vi "SumTwoh.vi"(0 "h1":dbl[](array[numeric]) format="%.2f", 1 "delay1":i32, 2 "h2":dbl[](array[numeric]) format="%.2f", 3 "delay2":i32) -> (4 "delay out":i32, 5 "upper":dbl[](array[numeric]) format="%.2f", 6 "h sum":dbl[](array[numeric]) format="%.2f", 7 "lower":dbl[](array[numeric]) format="%.2f")   [LabVIEW 2022 SP3]
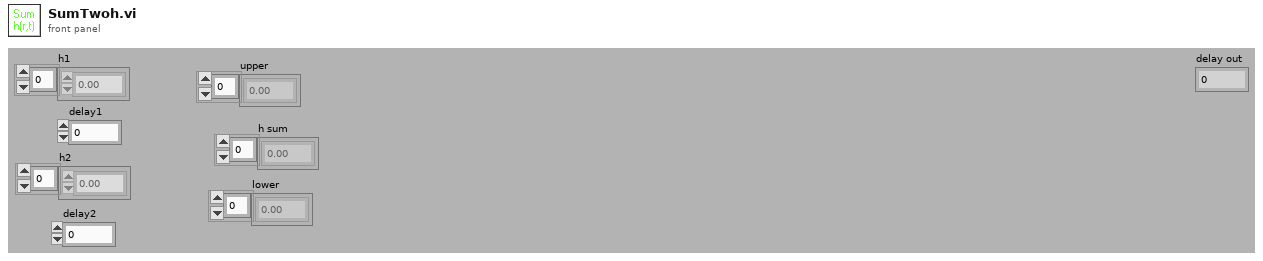
[diagram p1: front panel]
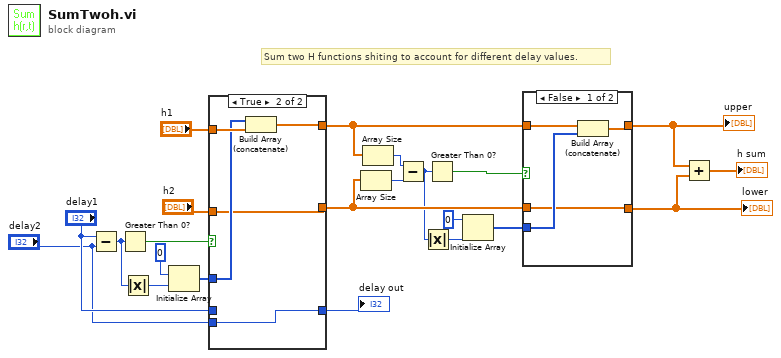
[diagram p0: block diagram]
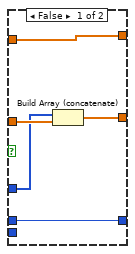
[diagram p2: hidden frame]
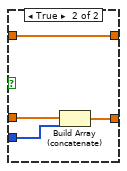
[diagram p3: hidden frame]
diagram:
  # "Sum two H functions shiting to account for different delay values."
  n1 = Subtract(x="delay1", y="delay2") -> (x-y=w2:i32)
  n2 = Greater Than 0?(x=w2) -> (x > 0?=w1:bool)
  n3 = Absolute Value(x=w2) -> (abs(x)=w17:i32)
  n4 = Initialize Array(0, w17) -> (w5:i32[])
  n5 = case shown="True" w1 {
    tunnel: "h1" -> [w25 w32]
    tunnel: "h2" -> [w27 w28]
    tunnel: [w23 w31] -> w4
    tunnel: "delay2" -> [_ w31]
    tunnel: w5 -> [w26 w30]
    tunnel: [w25 w29] -> w13
    tunnel: [w24 w28] -> w21
    tunnel: "delay1" -> [w23 _]
    frame False {
      n6 = Build Array (concatenate)(w26, w27) -> (w24:dbl[])
    }
    frame True {
      n7 = Build Array (concatenate)(w30, w32) -> (w29:dbl[])
    }
  }
  "delay out" <- w4
  n8 = Array Size(array=w21) -> (size(s)=w8:i32)
  n9 = Array Size(array=w13) -> (size(s)=w7:i32)
  n10 = Subtract(x=w7, y=w8) -> (x-y=w10:i32)
  n11 = Absolute Value(x=w10) -> (abs(x)=w15:i32)
  n12 = Greater Than 0?(x=w10) -> (x > 0?=w9:bool)
  n13 = Initialize Array(0, w15) -> (w11:i32[])
  n14 = case shown="False" w9 {
    tunnel: w13 -> [w36 w38]
    tunnel: w11 -> [w35 w39]
    tunnel: w21 -> [w33 w40]
    tunnel: [w34 w38] -> w20
    tunnel: [w33 w37] -> w22
    frame False {
      n15 = Build Array (concatenate)(w36, w35) -> (w34:dbl[])
    }
    frame True {
      n16 = Build Array (concatenate)(w40, w39) -> (w37:dbl[])
    }
  }
  "lower" <- w22
  "upper" <- w20
  n17 = Add(x=w20, y=w22) -> (x+y=→"h sum":dbl[])
